vi "Create DblArrayMsg.vi"(8 "error in (no error)":errorcluster, 10 "Message Data":dbl[](array[numeric]), 11 "Message Name":string) -> (0 "error out":errorcluster, 3 "DblArrayMsg Out":refnum<class "DblArrayMsg.lvclass">)   [LabVIEW 2009, in "LapDog.Messaging.v2.NativeArrays.lvlib" / "DblArrayMsg.lvclass"]
doc: "Returns a DblArrayMsg object with the given name.\n\nThis method executes regardless of the error in state."
uses:
  DblArrayMsg.lvclass
  DblArrayMsg.lvclass/DblArrayMsg.ctl
  Messaging.v2/MessageObject/Message.lvclass
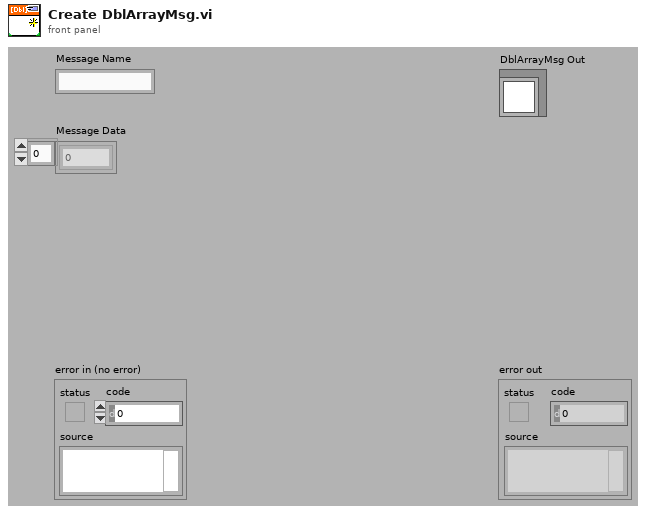
[diagram p1: front panel]
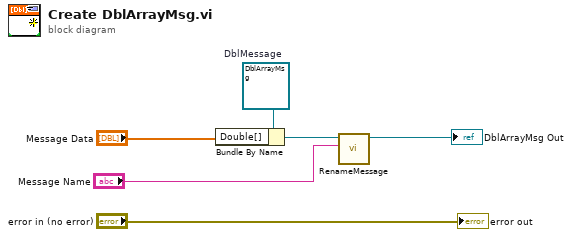
[diagram p0: block diagram]
diagram:
  w6 = refnum<class "DblArrayMsg.lvclass"> refnum  # DblMessage
  n1 = Bundle By Name(cluster=w6, "Double[]"="Message Data") -> (w3:refnum<class "DblArrayMsg.lvclass">)
  n2 = call "RenameMessage.vi"("Message Name"="Message Name", "Message in"=w3) -> ("Message out"=→"DblArrayMsg Out":refnum<class "DblArrayMsg.lvclass">)  [unwired: 8 in, 1 out]
  "error out" <- "error in (no error)"
